vi "get_triggerable_flag.vi"(8 "error in (no error)":errorcluster, 11 "GenericSignalReader in":refnum<class "GenericSignalReader.lvclass">) -> (0 "error out":errorcluster, 2 "triggerable?":bool, 3 "GenericSignalReader out":refnum<class "GenericSignalReader.lvclass">)   [LabVIEW 2010, in "GenericSignalReader.lvclass"]
uses:
  GenericSignalReader.lvclass
  GenericSignalReader.lvclass/GenericSignalReader.ctl
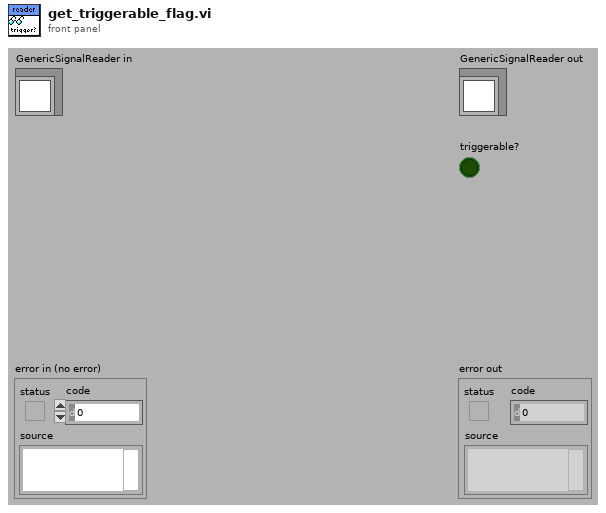
[diagram p1: front panel]
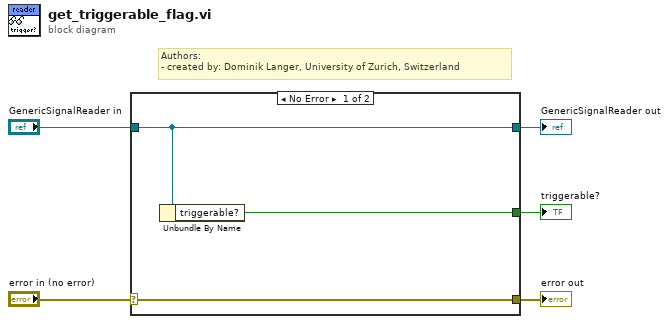
[diagram p0: block diagram]
diagram:
  # "Authors: \n- created by: Dominik Langer, University of Zurich, Switzerland"
  n1 = case shown="No Error" "error in (no error)" {
    selector: "error in (no error)" -> [w8 w9]
    tunnel: [w8 w9] -> w4
    tunnel: [w7 w10] -> w2
    tunnel: "GenericSignalReader in" -> [w7 w10]
    tunnel: [w6 _] -> w1
    frame No Error {
      n2 = Unbundle By Name(w7) -> ("triggerable?"=w6:bool)
    }
    frame Error {
    }
  }
  "error out" <- w4
  "GenericSignalReader out" <- w2
  "triggerable?" <- w1
